vi "Delete Memory.vi"(8 "Error In":errorcluster, 11 "Memory Object In":T1={"Device ID"=0, "Memeroy ID"=0, "Dimension"={"Depth"=1, "Height"=1, "Width"=1}, "Memory Type"=enum."32f"} {"Dimension"."Width" min=1; "Dimension"."Height" min=1; "Dimension"."Depth" min=1}) -> (0 "Error Out":errorcluster, 3 "Device Out":T2)   [LabVIEW 2012]
doc: "Deletes allocated memory on a device. It is best to call this at the end to avoid memory fragmentation due to constantly allocating and deleting memory."
uses:
  Non-User VIs/Controls/Device ID.ctl
  Non-User VIs/Controls/Memory Object.ctl
  Non-User VIs/Controls/Memory ID.ctl
  User Controls/Array Dimensions.ctl
  Non-User VIs/Controls/Memory Type.ctl
  Non-User VIs/Error Checking/Add Error Functional Global.vi
  OpenCLV x64.lvlib
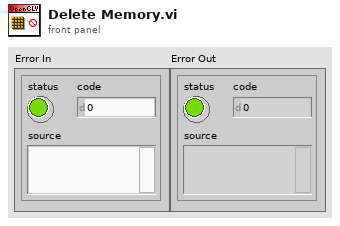
[diagram p1: front panel]
types:
  T1 = typedef "OpenCLV x64.lvlib/Memory Object.ctl" = cluster{"Device ID":T2, "Memeroy ID":T3, "Dimension":T4, "Memory Type":T5}
  T2 = typedef "OpenCLV x64.lvlib/Device ID.ctl" = u64
  T3 = typedef "OpenCLV x64.lvlib/Memory ID.ctl" = u64
  T4 = typedef "Array Dimensions.ctl" = cluster{"Depth":u64, "Height":u64, "Width":u64}
  T5 = typedef "OpenCLV x64.lvlib/Memory Type.ctl" = enum16{"32f", "u8", "i8", "u16", "i16", "u32", "i32", "64f"}
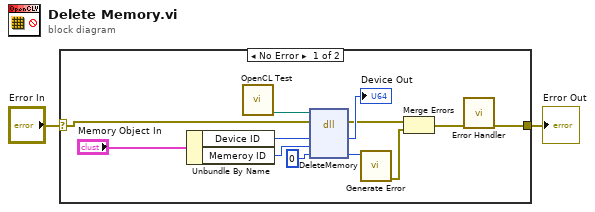
[diagram p0: block diagram]
diagram:
  n1 = case shown="No Error" "Error In" {
    selector: "Error In" -> [w3 w15]
    tunnel: [w7 w15] -> w1
    frame No Error {
      n2 = Unbundle By Name("Memory Object In") -> ("Device ID"=w11:T2, "Memeroy ID"=w12:T3)
      n3 = call "OpenCL Test.vi"() -> ("DLL To Use"=w8:path)  [unwired: 11 in]
      n4 = dll-call lib="C:/Users/bme-amcelroy-la/Desktop/OpenCLV/trunk/OpenCLV_x64_1.0/OpenCLV_x64.dll" fn="DeleteMemory"(path in=w8, error in=w3, "Device"=w11, "Device Memory"=w12, "Error"=0) -> (error out=w4:errorcluster, "Device"=→"Device Out":u64, "Error"=w13:i32)  [unwired: 3 in, 1 out]
      n5 = call "Generate Error.vi"("Error"=w13) -> ("error out"=w6:errorcluster)  [unwired: 10 in]
      n6 = Merge Errors(w4, w6) -> (w5:errorcluster)
      n7 = call-poly "Error Handler.vi"("Error In"=w5) -> ("Error Out"=w7:errorcluster)  [unwired: 10 in]
    }
    frame Error {
    }
  }
  "Error Out" <- w1
